vi "GlobalElevator.vi"() -> ()   [LabVIEW 2023]
panel:
  out "OUT_Elevator_Has_Arrived":bool
  out "OUT_Climbed":bool
  in  "SEN_Elevator_(in)":dbl
  in  "OUT_Elevator_PID_Mode":enum16{"Safety", "Travelling", "Positioning"}(ring)
  in  "OUT_Elevator_Left":dbl
  in  "OUT_Elevator_Right_(in)":dbl
  in  "REF_Elevator_Left":string
  in  "REF_Elevator_Right":string
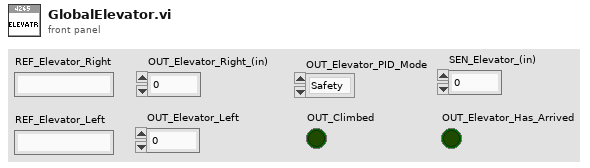
[diagram p1: front panel]
diagram:
